vi "intento de pajarera 2.vi"() -> ()   [LabVIEW 2014]
uses:
  Instance           4 18Saved   graph temp .vi
panel:
  in  "RESOL CH1 2":dbl
  in  "RANGE CH1 (V) 2":dbl=0.1
  out "temp 2":ext[](array[numeric]) format="%#_10e"
  out "R(temp) 2":ext(graph)
  in  "Mult Temp baño 2":u16(ring)=1 items=["3458", "34420", "34401"]
  in  "addrss instr 2  (board addrs:instrum addrs) 2":string="0:13"
  out "adrs temp baño \n(board addrs:instrum addrs) 2":string="0:6"
  in  "addrss instr 1  (board addrs:instrum addrs)":string="0:14"
  out "R(temp)":ext(graph)
  out "temp":ext[](array[numeric]) format="%#_10e"
  in  "File Name":path=path "C:/Users/INTI/Desktop/Gonzalo/mediciones"
  in  "stop":bool
  out "adrs temp baño \n(board addrs:instrum addrs)":string="0:6"
  in  "Mult Temp baño":u16(ring)=2 items=["3458", "34420", "34401"]
  # "Instrucciones\n1- seleccionar directorio y file name\n2- seleccione multimetro a utilizar y addrss\n2- play empieza a graficar y grabar medidas\n3- stop, finaliza (mantener apretado)"
  # "MEDICION TEMP CON 3458"
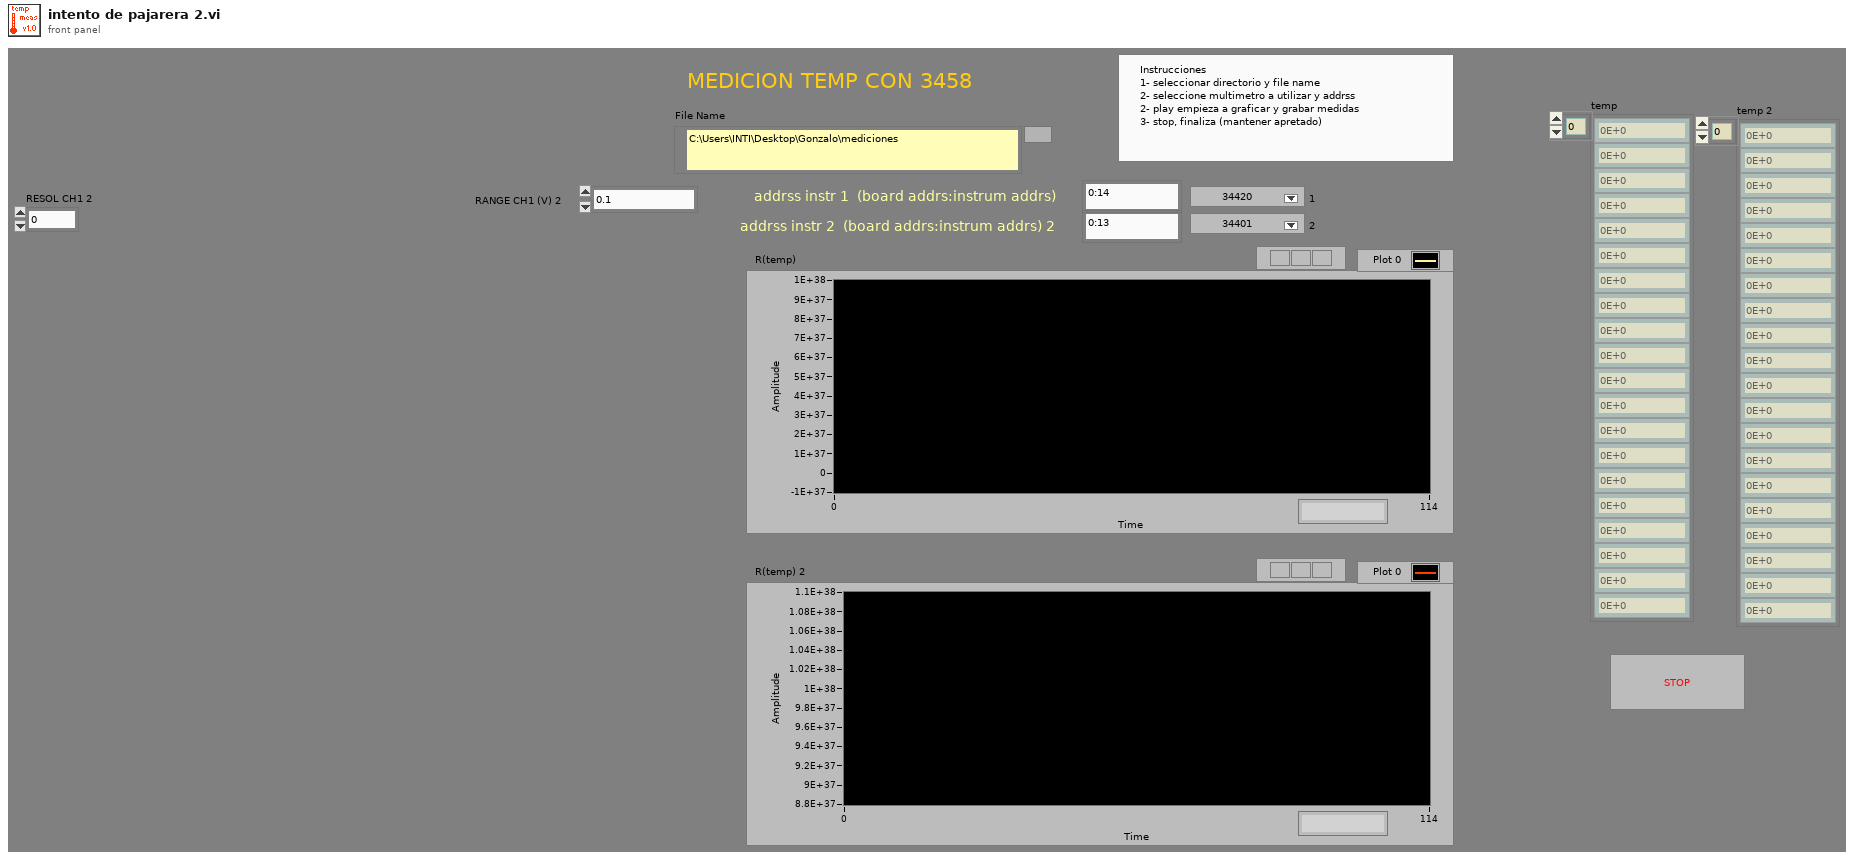
[diagram p1: front panel]
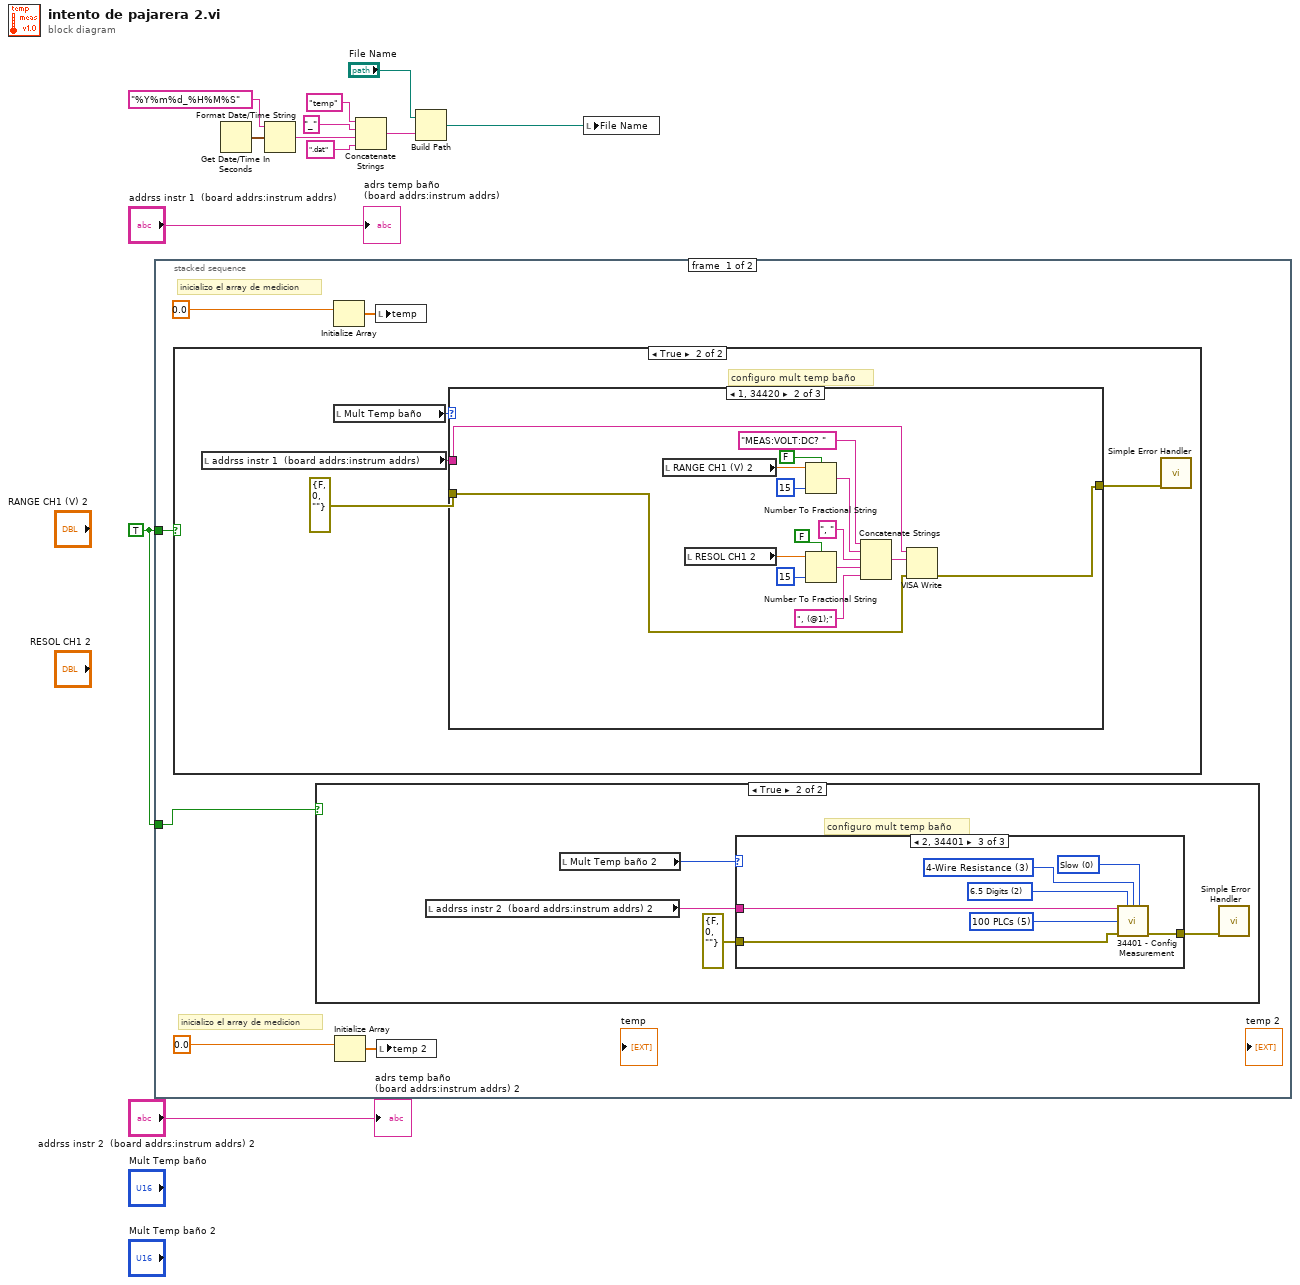
[diagram p0: block diagram]
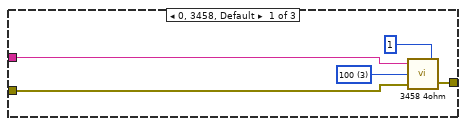
[diagram p3: hidden frame]
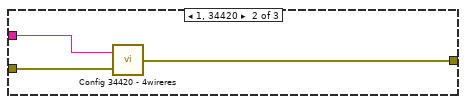
[diagram p4: hidden frame]
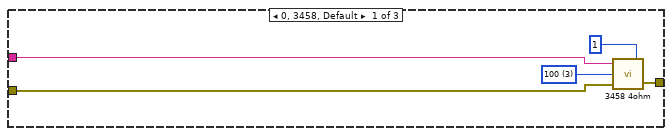
[diagram p6: hidden frame]
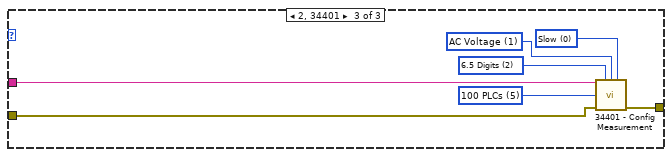
[diagram p7: hidden frame]
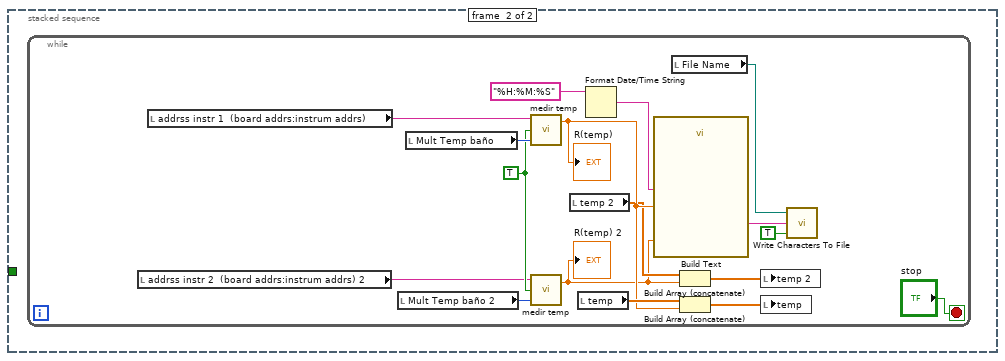
[diagram p8: hidden frame]
diagram:
  w1 = TRUE
  n1 = stacked-sequence {
    tunnel: w1 -> [w16 _]
    tunnel: w1 -> [w15 _]
    frame #0 {
      # "inicializo el array de medicion"
      # "inicializo el array de medicion"
      n2 = case shown="True" w16 {
        frame False {
        }
        frame True {
          # "configuro mult temp baño"
          n3 = local read "addrss instr 1  (board addrs:instrum addrs)"() -> (w40:string)
          n4 = local read "Mult Temp baño"() -> (w41:u16)
          n5 = case shown="1, 34420" w41 {
            tunnel: w40 -> [w45 w48 w64]
            tunnel: errorcluster {"status"=FALSE, "code"=0, "source"=""} ("error OUT 2") -> [w46 w47 w63]
            tunnel: [w42 w49 w62] -> w38
            frame 0, 3458, Default {
              w43 = u16 3 items=["10", "20", "50", "100", "200"] ("NPLC")
              n6 = call "3458 4ohm.vi"("NRDGS"=1, "error in (no error)"=w46, "NPLC"=w43, "Multímetro TRP"=w45) -> ("error out"=w42:errorcluster)
            }
            frame 1, 34420 {
              n7 = local read "RANGE CH1 (V) 2"() -> (w60:dbl)
              n8 = local read "RESOL CH1 2"() -> (w55:dbl)
              n9 = Number To Fractional String(use system decimal point (T)=FALSE, number=w60, precision (6)=i16 15) -> (F-format string=w58:string)  [unwired: 1 in]
              n10 = Number To Fractional String(use system decimal point (T)=FALSE, number=w55, precision (6)=i16 15) -> (F-format string=w54:string)  [unwired: 1 in]
              n11 = Concatenate Strings("MEAS:VOLT:DC? " ("write buffer"), w58, ", " ("string"), w54, ", (@1);" ("string")) -> (w52:string)
              n12 = VISA Write(VISA resource name=w48, write buffer=w52, error in (no error)=w47) -> (error out=w49:errorcluster)  [unwired: 2 out]
            }
            frame 2, 34401 {
              w68 = u16 5 items=["Default", "0.02 PLCs", "0.2 PLC", "1 PLCs", "10 PLCs", "100 PLCs"] ("Manual Int. (0:Default)")
              w67 = u16 0 items=["Slow", "Medium", "Fast"] ("AC Filter (1:Medium)")
              w66 = u16 1 items=["DC Voltage", "AC Voltage", "2--Wire Resistance", "4-Wire Resistance", "DC Current", "AC Current", "Frequency", "Period", "Continuity", "Diode Checking", "VDC: VDC Ratio"] ("Function (0:V DC)")
              w65 = u16 2 items=["4.5 Digits", "5.5 Digits", "6.5 Digits"] ("Manual Res. (1:5.5 Digits)")
              n13 = call "34401 - Config Measurement.vi"("address"=w64, "Manual Res. (1:5.5 Digits)"=w65, "Function (0:V DC)"=w66, "AC Filter (1:Medium)"=w67, "Manual Int. (0:Default)"=w68, "error in (no error)"=w63) -> ("error out"=w62:errorcluster)  [unwired: 9 in]
            }
          }
          n14 = call <vilib>:"Simple Error Handler.vi"("error in (no error)"=w38) -> ()  [unwired: 4 in, 5 out]
        }
      }
      n15 = case shown="True" w15 {
        frame False {
        }
        frame True {
          # "configuro mult temp baño"
          n16 = local read "addrss instr 2  (board addrs:instrum addrs) 2"() -> (w21:string)
          n17 = local read "Mult Temp baño 2"() -> (w22:u16)
          n18 = case shown="2, 34401" w22 {
            tunnel: w21 -> [w26 w30 w33]
            tunnel: errorcluster {"status"=FALSE, "code"=0, "source"=""} ("error OUT 2") -> [w27 w29 w32]
            tunnel: [w23 w28 w31] -> w19
            frame 0, 3458, Default {
              w24 = u16 3 items=["10", "20", "50", "100", "200"] ("NPLC")
              n19 = call "3458 4ohm.vi"("NRDGS"=1, "error in (no error)"=w27, "NPLC"=w24, "Multímetro TRP"=w26) -> ("error out"=w23:errorcluster)
            }
            frame 1, 34420 {
              n20 = call "Config 34420 - 4wireres.vi"("error IN"=w29, "Address 34420 (default: 13)"=w30) -> ("error out"=w28:errorcluster)
            }
            frame 2, 34401 {
              w37 = u16 5 items=["Default", "0.02 PLCs", "0.2 PLC", "1 PLCs", "10 PLCs", "100 PLCs"] ("Manual Int. (0:Default)")
              w36 = u16 0 items=["Slow", "Medium", "Fast"] ("AC Filter (1:Medium)")
              w35 = u16 3 items=["DC Voltage", "AC Voltage", "2--Wire Resistance", "4-Wire Resistance", "DC Current", "AC Current", "Frequency", "Period", "Continuity", "Diode Checking", "VDC: VDC Ratio"] ("Function (0:V DC)")
              w34 = u16 2 items=["4.5 Digits", "5.5 Digits", "6.5 Digits"] ("Manual Res. (1:5.5 Digits)")
              n21 = call "34401 - Config Measurement.vi"("address"=w33, "Manual Res. (1:5.5 Digits)"=w34, "Function (0:V DC)"=w35, "AC Filter (1:Medium)"=w36, "Manual Int. (0:Default)"=w37, "error in (no error)"=w32) -> ("error out"=w31:errorcluster)  [unwired: 9 in]
            }
          }
          n22 = call <vilib>:"Simple Error Handler.vi"("error in (no error)"=w19) -> ()  [unwired: 4 in, 5 out]
        }
      }
      n23 = Initialize Array(0.0 ("element")) -> (w17:dbl[])  [unwired: 1 in]
      n24 = Initialize Array(0.0 ("element")) -> (w14:dbl[])  [unwired: 1 in]
      n25 = local write "temp"(w17) -> ()
      n26 = local write "temp 2"(w14) -> ()
    }
    frame #1 {
      n27 = while {
        stop <- "stop" stop-if-true
        w72 = TRUE ("Medir Temperatura")
        n28 = local read "addrss instr 2  (board addrs:instrum addrs) 2"() -> (w71:string)
        n29 = local read "addrss instr 1  (board addrs:instrum addrs)"() -> (w84:string)
        n30 = local read "Mult Temp baño 2"() -> (w70:u16)
        n31 = local read "Mult Temp baño"() -> (w85:u16)
        n32 = call "medir temp.vi"("multimetro"=w85, "Medir Temperatura"=w72, "address string"=w84) -> ("Numeric"=w76:ext)  [unwired: 1 in]
        "R(temp)" <- w76
        n33 = call "medir temp.vi"("multimetro"=w70, "Medir Temperatura"=w72, "address string"=w71) -> ("Numeric"=w69:ext)  [unwired: 1 in]
        "R(temp) 2" <- w69
        n34 = local read "temp 2"() -> (w74:ext[])
        n35 = local read "temp"() -> (w79:ext[])
        n36 = Format Date/Time String(time format string (%c)="%H:%M:%S") -> (date/time string=w80:string)  [unwired: 2 in]
        n37 = call "Build Text"("tiempo"=w80, "Temp Multimetro 1"=w76, "Temp Multimetro 2"=w69) -> ("Result"=w82:string)  [unwired: 11 in, 1 out]
        n38 = local read "File Name"() -> (w75:path)
        n39 = Build Array (concatenate)(w74, w69) -> (w73:ext[])
        n40 = Build Array (concatenate)(w79, w76) -> (w77:ext[])
        n41 = local write "temp 2"(w73) -> ()
        n42 = local write "temp"(w77) -> ()
        n43 = call <vilib>:"Write Characters To File.vi"("append to file? (new file:F)"=TRUE, "character string"=w82, "file path (dialog if empty)"=w75) -> ()  [unwired: 2 in, 1 out]
      }
    }
  }
  n44 = Get Date/Time In Seconds() -> (seconds since 1Jan1904=w5:timestamp)
  n45 = Format Date/Time String(time format string (%c)="%Y%m%d_%H%M%S", seconds (now)=w5) -> (date/time string=w3:string)  [unwired: 1 in]
  n46 = Concatenate Strings("temp" ("string"), "_" ("string"), w3, ".dat" ("string")) -> (w7:string)
  n47 = Build Path(base path="File Name", name or relative path=w7) -> (appended path=w6:path)
  n48 = local write "File Name"(w6) -> ()
  "adrs temp baño \n(board addrs:instrum addrs)" <- "addrss instr 1  (board addrs:instrum addrs)"
  "adrs temp baño \n(board addrs:instrum addrs) 2" <- "addrss instr 2  (board addrs:instrum addrs) 2"
